vi "CreateHeader.vi"(7 "WPILOG_Version":i16=1, 11 "extra header string":string) -> (3 "header":u8[](array[numeric]) format="%x")   [LabVIEW 2023]
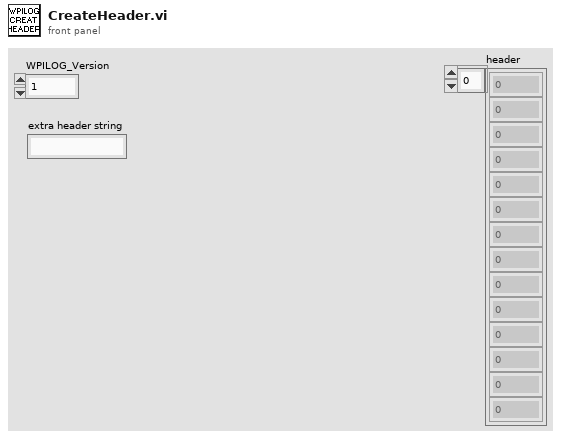
[diagram p1: front panel]
types:
  T1 = enum16{"big-endian, network order", "native, host order", "little-endian"}
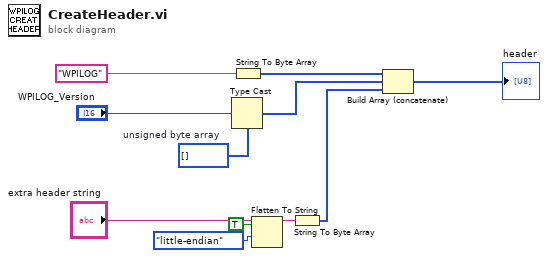
[diagram p0: block diagram]
diagram:
  w11 = u8[] []  # unsigned byte array
  n1 = Type Cast(type=w11, x="WPILOG_Version") -> (*(type *) &x=w9:u8[])
  n2 = String To Byte Array(string="WPILOG") -> (unsigned byte array=w10:u8[])
  n3 = Flatten To String(anything="extra header string", prepend array or string size? (T)=TRUE, byte order (0:big-endian, network order)=T1."little-endian") -> (data string=w4:string)  [unwired: 1 in, 2 out]
  n4 = String To Byte Array(string=w4) -> (unsigned byte array=w2:u8[])
  n5 = Build Array (concatenate)(w10, w9, w2) -> (→"header":u8[])
